vi "Launch.vi"(8 "error in (no error)":errorcluster) -> (0 "error out":errorcluster, 3 "Actor API out":refnum<class "Actor API.lvclass">)   [LabVIEW 2015, in "About Window.lvclass"]
doc: "<b>Response</b> channel is used by this actor to return infomation back to the parent. Typically this input is the Request channel of the parent actor."
uses:
  About Window.lvclass
  Re-use Libraries/Minimal Actor Framework/Actors/Base Actor/API/Actor API.lvclass
  Re-use Libraries/Minimal Actor Framework/Actors/Base Actor/Actor/Front Panel State.ctl
  Re-use Libraries/Minimal Actor Framework/Messaging/Messenger/Messenger.lvclass
  Re-use Libraries/Minimal Actor Framework/Actors/Base Actor/Actor/Actor.lvclass/Actor.ctl
  Re-use Libraries/Minimal Actor Framework/Actors/Base Actor/Actor/Actor.lvclass
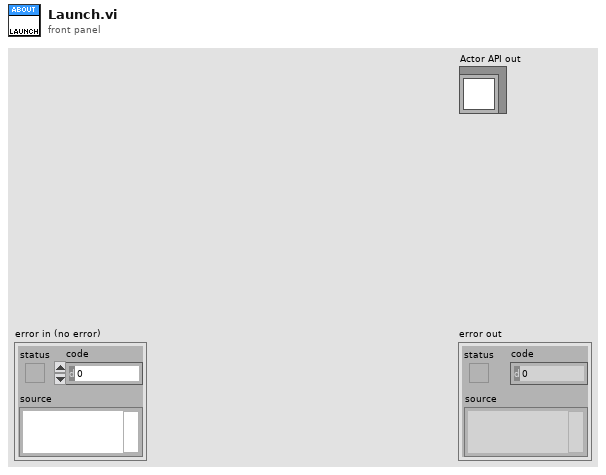
[diagram p1: front panel]
types:
  T1 = typedef "Actor.lvclass/Front Panel State.ctl" = enum32{"Invalid", "Standard", "Closed", "Hidden", "Minimized", "Maximized"}
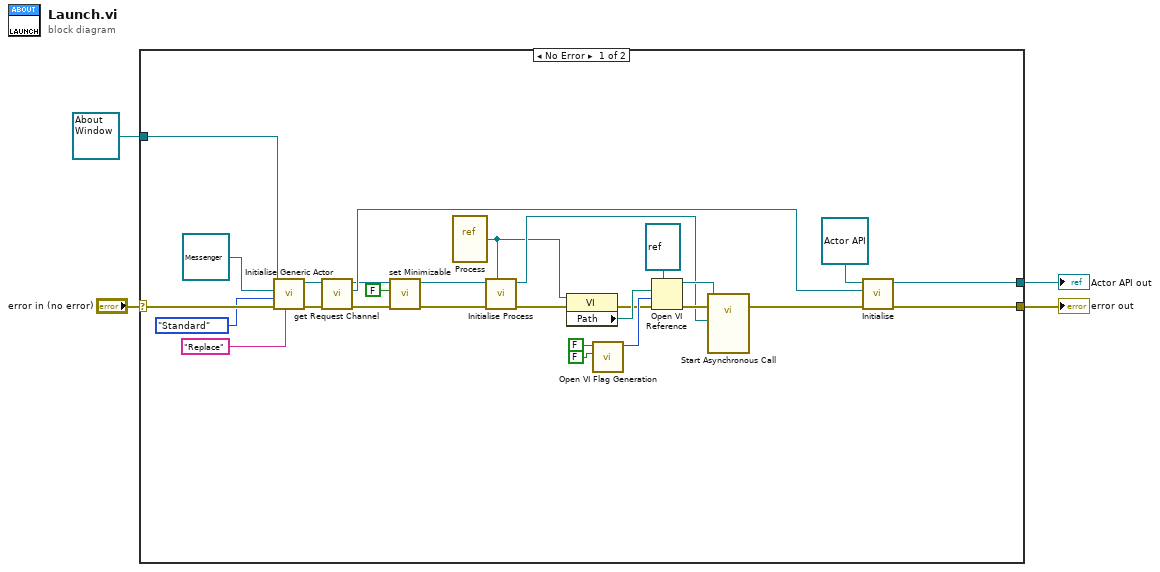
[diagram p0: block diagram]
diagram:
  n1 = case shown="No Error" "error in (no error)" {
    selector: "error in (no error)" -> [w23 w32]
    tunnel: [w20 w32] -> w4
    tunnel: [w13 _] -> w1
    tunnel: refnum<class "About Window.lvclass"> refnum ("Worker Test 1.lvclass") -> [w22 _]
    frame No Error {
      n2 = call-dynamic "Initialise Generic Actor.vi"("Name"="Replace", "Front Panel State"=Front_Panel_State."Standard", "Response Channel"=refnum<class "Messenger.lvclass"> refnum, "Actor in"=w22) -> ("Actor out"=w24:refnum<class "About Window.lvclass">)  [unwired: 6 in, 1 out]
      n3 = call "get Request Channel.vi"("error in (no error)"=w23, "Actor in"=w24) -> ("error out"=w9:errorcluster, "Request Channel"=w25:refnum<class "Messenger.lvclass">, "Actor out"=w10:refnum<class "About Window.lvclass">)  [unwired: 7 in]
      n4 = call "set Minimizable.vi"("error in (no error)"=w9, "Minimizable"=FALSE, "Actor in"=w10) -> ("error out"=w7:errorcluster, "Actor out"=w8:refnum<class "About Window.lvclass">)  [unwired: 7 in]
      n5 = vi-ref "Process.vi"() -> (w14:refnum<vi>)
      n6 = call-dynamic "Initialise Process.vi"("Process"=w14, "error in (no error)"=w7, "Actor in"=w8) -> ("error out"=w15:errorcluster, "Actor out"=w16:refnum<class "About Window.lvclass">)  [unwired: 7 in]
      n7 = property class="VI"(reference=w14, error in=w15) -> (error out=w18:errorcluster, "Path"=w19:path)  [unwired: 1 out]
      n8 = call "Open VI Flag Generation.vi"("Call And Collect (F)"=FALSE, "Re-entrant (F)"=FALSE) -> ("Flags"=w31:i32)  [unwired: 9 in]
      n9 = Open VI Reference(type specifier VI Refnum (for type only)=refnum<vi> refnum, vi path=w19, options=w31, error in (no error)=w18) -> (vi reference=w27:refnum<vi>, error out=w26:errorcluster)  [unwired: 2 in]
      n10 = call-by-ref "Start Asynchronous Call"(reference=w27, error in=w26, "Worker Test 1.lvclass"=w16) -> (error out=w11:errorcluster)  [unwired: 11 in, 1 out]
      n11 = call "Initialise.vi"("error in (no error)"=w11, "Request Channel"=w25, "Actor API in"=refnum<class "Actor API.lvclass"> refnum ("Actor API.lvclass")) -> ("error out"=w20:errorcluster, "Actor API out"=w13:refnum<class "Actor API.lvclass">)  [unwired: 7 in]
    }
    frame Error {
    }
  }
  "error out" <- w4
  "Actor API out" <- w1
